vi "OnshapeTwin.vi"(7 "JPG":refnum<vi>, 10 "queueName":string="PV_script", 11 "Console Reference":refnum<vi>) -> ()   [LabVIEW 2024]
uses:
  arm/onshape/Onshape/ReadOnshapeAngle.vi
  arm/onshape/Onshape/WriteOnshapeAngle.vi
  <vilib>/Platform/browser.llb/Open URL in Default Browser (string).vi
panel:
  in  "open":bool
  in  "URL":string="https://cad.onshape.com/documents/357307b443615149a777ac6d/w/b0d2bfb6c7a5e8be1349caee/e/a0c2ded96ad1358661334f7b"
  in  "Mode":T1(tab)=enum."No Control"
  out "Init code":string="import hub,time\n\nupper = hub.port.A.motor\nlower = hub.port.E.motor\nlower.mode(1)\nupper.mode(1)\nlower.brake()\nupper.brake()\n"
  out "shoulder":dbl(slide)=43.24022346368716 scale=-180.0..180.0
  out "elbow":dbl(slide)=137.76536312849163 scale=-180.0..180.0
  out "cmds sent":string
  out "New Line":string
  out "elbow 2":dbl(slide)=137.76536312849163 scale=-180.0..180.0
  out "shoulder 2":dbl(slide)=43.24022346368716 scale=-180.0..180.0
  in  "Ctrl C":bool
  in  "start":bool
  in  "python":string
  in  "Send":bool
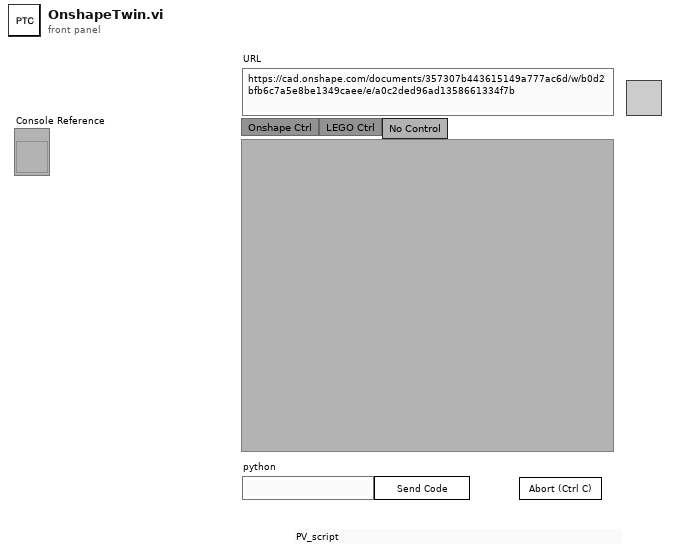
[diagram p1: front panel]
types:
  T1 = enum32{"Onshape Ctrl", "LEGO Ctrl", "No Control"}
  T2 = cluster{"URL":string, "URL":string, "URL":string}
  T3 = enum16{"Not data", "single values", "XY pairs", "Arrays", "Matrix"}
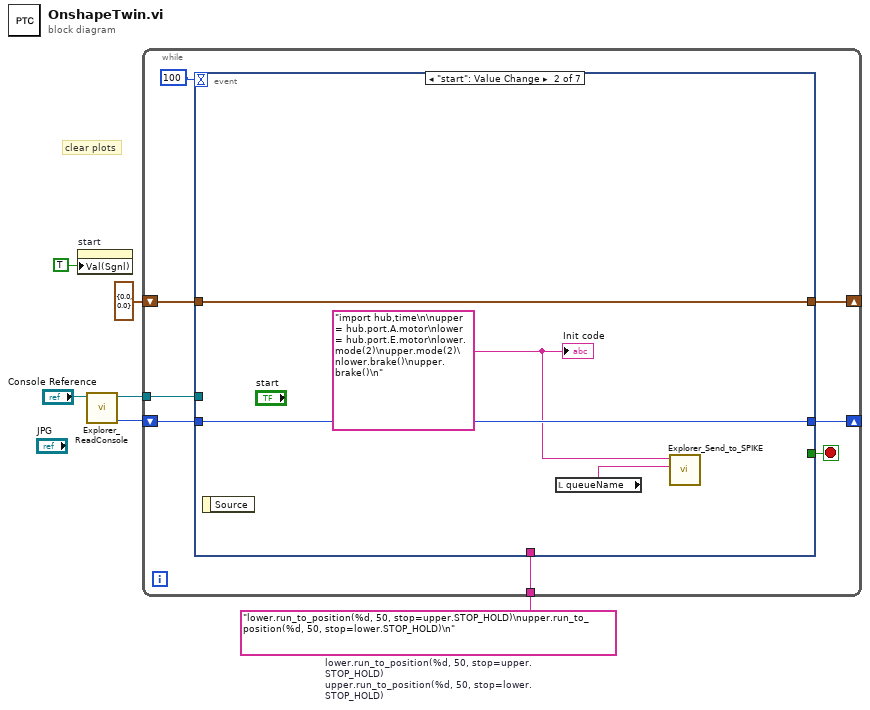
[diagram p0: block diagram]
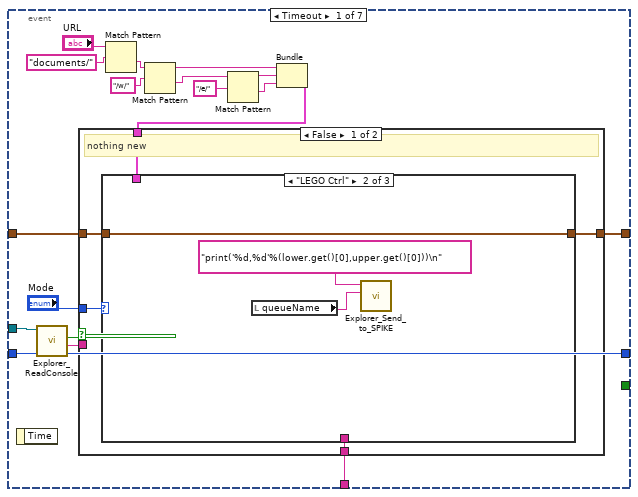
[diagram p2: hidden frame]
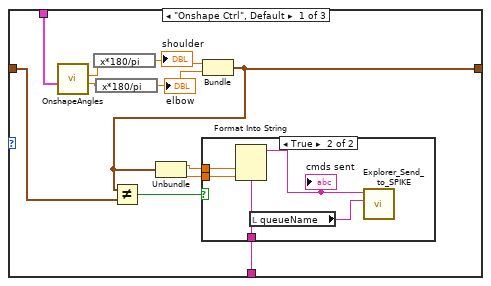
[diagram p3: hidden frame]
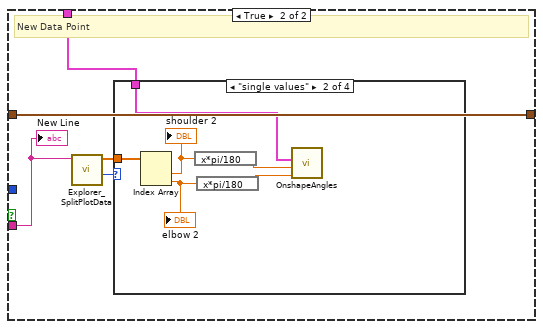
[diagram p6: hidden frame]
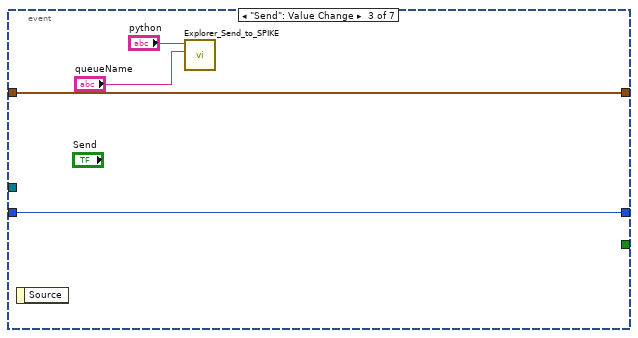
[diagram p10: hidden frame]
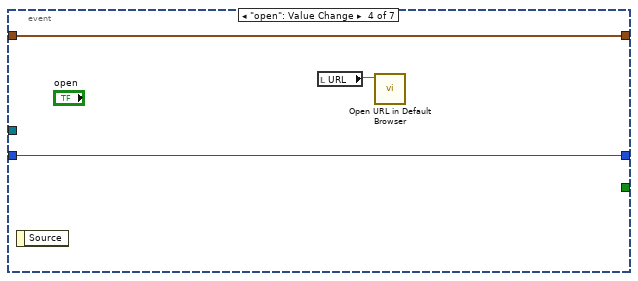
[diagram p11: hidden frame]
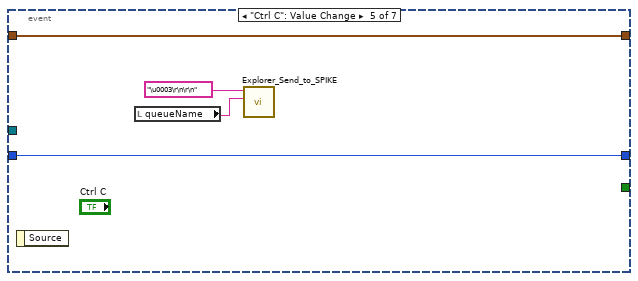
[diagram p12: hidden frame]
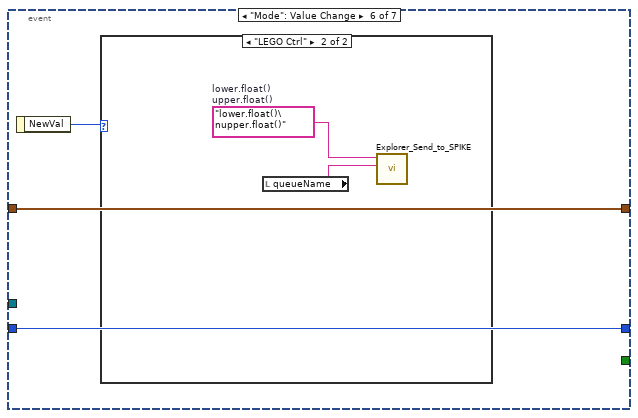
[diagram p13: hidden frame]
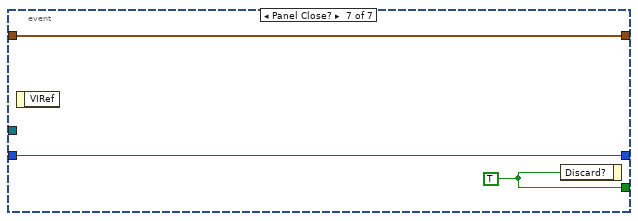
[diagram p15: hidden frame]
diagram:
  w1 = "lower.run_to_position(%d, 50, stop=upper.STOP_HOLD)\nupper.run_to_position(%d, 50, stop=lower.STOP_HOLD)\n"  # lower.run_to_position(%d, 50, stop=upper.STOP_HOLD) upper.run_to_position(%d, 50, stop=lower.STOP_HOLD)
  # "clear plots"
  n1 = property on="start" class="Bool (strict)"("Val(Sgnl)"=TRUE ("Value (Signaling)")) -> ()  [unwired: 2 in, 2 out]
  n2 = call "Explorer_ReadConsole.vi"("String in"="Console Reference") -> ("index out"=w5:i32, "String out"=w4:refnum<vi>)  [unwired: 6 in, 3 out]
  n3 = while {
    shift-right: [w12] -> _
    shift-left: w5 -> [w11]
    tunnel: w4 -> [w10]
    shift-right: [w9] -> _
    shift-left: cluster{"Angle1Out":dbl, "Angle2Out":dbl} {"Angle1Out"=0.0, "Angle2Out"=0.0} -> [w8]
    tunnel: w1 -> [w7]
    stop <- w13 stop-if-true
    n4 = event shown="[1] \"start\": Value Change" {
      selector: _ -> [_ _ _ _ _ _ _]
      dyn-events: _ -> [_ _ _ _ _ _ _]
      timeout: 100 -> [_ _ _ _ _ _ _]
      tunnel: [_ _ _ _ _ _ w92] -> w13
      tunnel: [w32 w73 w77 w80 w84 w86 w91] -> w12
      tunnel: w11 -> [w33 w73 w77 w80 w84 w86 w91]
      tunnel: w10 -> [w29 _ _ _ _ _ _]
      tunnel: [w28 w72 w74 w79 w81 w87 w90] -> w9
      tunnel: w8 -> [w27 w72 w74 w79 w81 w87 w90]
      tunnel: w7 -> [w26 _ _ _ _ _ _]
      event Timeout {
        n5 = event-data() -> ()  [unwired: 1 in, 1 out]
        n6 = call "Explorer_ReadConsole.vi"("index in"=w33, "String in"=w29) -> ("index out"=w32:i32, "New Line"=w31:string, "New point?"=w30:bool)  [unwired: 5 in, 2 out]
        n7 = Match Pattern(string="URL", regular expression="documents/") -> (after substring=w19:string)  [unwired: 1 in, 3 out]
        n8 = Match Pattern(string=w19, regular expression="/w/") -> (before substring=w21:string, after substring=w20:string)  [unwired: 1 in, 2 out]
        n9 = Match Pattern(string=w20, regular expression="/e/") -> (before substring=w22:string, after substring=w23:string)  [unwired: 1 in, 2 out]
        n10 = Bundle("URL"=w21, "URL"=w22, "URL"=w23) -> (w15:T2)  [unwired: 1 in]
        n11 = case shown="False" w30 {
          tunnel: w31 -> [_ w63]
          tunnel: [w36 w60] -> w28
          tunnel: w27 -> [w38 w60]
          tunnel: w26 -> [w37 _]
          tunnel: "Mode" -> [w35 _]
          tunnel: w15 -> [w34 w59]
          frame False {
            # "nothing new"
            n12 = case shown="\"LEGO Ctrl\"" w35 {
              tunnel: w38 -> [w45 w57 w58]
              tunnel: w37 -> [w43 _ _]
              tunnel: [w42 w57 w58] -> w36
              tunnel: w34 -> [w39 _ _]
              frame "Onshape Ctrl", Default {
                n13 = call-poly "OnshapeAngles.vi"("IDs"=w39) -> ("Angle2Out"=w47:dbl, "Angle1Out"=w46:dbl)  [unwired: 7 in, 2 out]
                n14 = expression code="x*180/pi"(w46) -> (w48:dbl)
                "shoulder" <- w48
                n15 = expression code="x*180/pi"(w47) -> (w49:dbl)
                "elbow" <- w49
                n16 = Bundle("Angle1Out"=w48, "Angle2Out"=w49) -> (w42:cluster{"Angle1Out":dbl, "Angle2Out":dbl})  [unwired: 1 in]
                n17 = Not Equal?(x=w42, y=w45) -> (x != y?=w44:bool)
                n18 = Unbundle(w42) -> ("Angle1Out"=w41:dbl, "Angle2Out"=w40:dbl)
                n19 = case shown="True" w44 {
                  tunnel: w43 -> [_ w53]
                  tunnel: w41 -> [_ w52]
                  tunnel: w40 -> [_ w51]
                  frame False {
                  }
                  frame True {
                    n20 = Format Into String(format string=w53, w52, w51) -> (resulting string=w50:string)  [unwired: 2 in, 1 out]
                    "cmds sent" <- w50
                    n21 = local read "queueName"() -> (w54:string)
                    n22 = call "Explorer_Send_to_SPIKE.vi"("queueName"=w54, "python"=w50) -> ()  [unwired: 9 in, 1 out]
                  }
                }
              }
              frame "LEGO Ctrl" {
                n23 = local read "queueName"() -> (w56:string)
                n24 = call "Explorer_Send_to_SPIKE.vi"("queueName"=w56, "python"="print('%d,%d'%(lower.get()[0],upper.get()[0]))\n") -> ()  [unwired: 9 in, 1 out]
              }
              frame "No Control" {
              }
            }
          }
          frame True {
            # "New Data Point"
            n25 = call "Explorer_SplitPlotData.vi"("Value"=w63) -> ("Data type"=w62:T3, "Array"=w61:dbl[])  [unwired: 8 in, 1 out]
            n26 = case shown="\"single values\"" w62 {
              tunnel: w61 -> [_ w69 _ _]
              tunnel: w59 -> [_ w64 _ _]
              frame Default {
              }
              frame "single values" {
                n27 = Index Array(array=w69) -> (element #1=w68:dbl, element #2=w67:dbl)  [unwired: 2 in]
                "elbow 2" <- w67
                "shoulder 2" <- w68
                n28 = expression code="x*pi/180"(w68) -> (w66:dbl)
                n29 = expression code="x*pi/180"(w67) -> (w65:dbl)
                n30 = call-poly "OnshapeAngles.vi"("Angle2In"=w65, "Angle1In"=w66, "IDs"=w64) -> ()  [unwired: 9 in]
              }
              frame "XY pairs" {
              }
              frame "Not data" {
              }
            }
            "New Line" <- w63
          }
        }
      }
      event "start": Value Change {
        w70 = "import hub,time\n\nupper = hub.port.A.motor\nlower = hub.port.E.motor\nlower.mode(2)\nupper.mode(2)\nlower.brake()\nupper.brake()\n" ("String")
        n31 = event-data() -> ()  [unwired: 1 in, 1 out]
        n32 = local read "queueName"() -> (w71:string)
        n33 = call "Explorer_Send_to_SPIKE.vi"("queueName"=w71, "python"=w70) -> ()  [unwired: 9 in, 1 out]
        "Init code" <- w70
      }
      event "Send": Value Change {
        n34 = event-data() -> ()  [unwired: 1 in, 1 out]
        n35 = call "Explorer_Send_to_SPIKE.vi"("queueName"="queueName", "python"="python") -> ()  [unwired: 9 in, 1 out]
      }
      event "open": Value Change {
        n36 = event-data() -> ()  [unwired: 1 in, 1 out]
        n37 = local read "URL"() -> (w78:string)
        n38 = call-poly <vilib>:"Open URL in Default Browser.vi"("URL"=w78) -> ()  [unwired: 5 in, 2 out]
      }
      event "Ctrl C": Value Change {
        n39 = event-data() -> ()  [unwired: 1 in, 1 out]
        n40 = local read "queueName"() -> (w82:string)
        n41 = call "Explorer_Send_to_SPIKE.vi"("queueName"=w82, "python"="\u0003\r\n\r\n" ("function name")) -> ()  [unwired: 9 in, 1 out]
      }
      event "Mode": Value Change {
        n42 = event-data() -> ("NewVal"=w85:T1)  [unwired: 1 in]
        n43 = case shown="\"LEGO Ctrl\"" w85 {
          frame "Onshape Ctrl", Default {
          }
          frame "LEGO Ctrl" {
            w88 = "lower.float()\nupper.float()"  # lower.float() upper.float()
            n44 = local read "queueName"() -> (w89:string)
            n45 = call "Explorer_Send_to_SPIKE.vi"("queueName"=w89, "python"=w88) -> ()  [unwired: 9 in, 1 out]
          }
        }
      }
      event Panel Close? {
        w92 = TRUE ("Discard?")
        n46 = event-data() -> ()  [unwired: 1 in, 1 out]
        n47 = event-data("Discard?"=w92) -> ()  [unwired: 1 in, 1 out]
      }
    }
  }
